vi "Test List Folder.vi"(8 "error in (no error)":errorcluster) -> (0 "error out":errorcluster, 3 "Pass?":bool)   [LabVIEW 2020]
uses:
  G-Unicode/Types/UTF-8 String/UTF-8 String.lvclass
  G-Unicode/Types/UTF-8 String/UTF-8 String.lvclass/UTF-8 String.ctl
  G-Unicode/Types/UTF-8 Path/UTF-8 Path.lvclass/UTF-8 Path.ctl
  a54f53b9-e182-45f2-9df3-3ad09404b159.vi
  2400d2f7-f357-4396-a7fa-e5c669c64687.vi
  2b28c85d-6eb6-42f1-9791-7ceb4d579ff7.vi
  8ef4e441-2967-427c-b2f5-611982e59b74.vi
  d10c2814-85e2-4189-8dec-6298f27de2e3.vi
  570365af-4a81-404b-8e59-15630106fe67.vi
  eeafece5-71ef-472f-ba41-926d6844275a.vi
  410ed48b-bd58-4d2b-973d-16e07af476d5.vi
  G-Unicode/Private/Conversion/Text as Encoded Path.vi
  G-Unicode/Private/Conversion/Polymorphic VIs/Text as Encoded Path (LabVIEW Path).vi
  G-Unicode/Types/UTF-8 Path/Write Encoded UTF-8 Path.vi
  G-Unicode/Private/Conversion/Path as Encoded Path.vi
  G-Unicode/Private/Conversion/Polymorphic VIs/Path as Encoded Path (LabVIEW Path).vi
  G-Unicode/Private/Conversion/Path as UTF-8 Path.vi
  G-Unicode/Private/Conversion/Polymorphic VIs/Path as UTF-8 Path (UTF-8 Path).vi
  2400d2f7-f357-4396-a7fa-e5c669c64687.vi/5269e09c-4216-478e-8686-9fb7d38e224a.vi
  2400d2f7-f357-4396-a7fa-e5c669c64687.vi/d1f4a45d-6f02-44dd-a40b-2b28d80e6519.vi
  G-Unicode/Private/Conversion/String as Encoded String.vi
  G-Unicode/Private/Conversion/Polymorphic VIs/String as Encoded String (UTF-8 String).vi
  G-Unicode/Private/Library/gu_list_folder.vi
  2400d2f7-f357-4396-a7fa-e5c669c64687.vi/8eb4f0ed-0012-4550-978e-be3f7301df70.vi
  2400d2f7-f357-4396-a7fa-e5c669c64687.vi/f7e6584c-01ed-423f-9bcd-660954191d0d.vi
  G-Unicode/Private/Conversion/Polymorphic VIs/Text as Encoded Path (UTF-8 String).vi
  G-Unicode/Private/Conversion/Polymorphic VIs/Path as Encoded Path (UTF-8 Path).vi
  8ef4e441-2967-427c-b2f5-611982e59b74.vi/5269e09c-4216-478e-8686-9fb7d38e224a.vi
  8ef4e441-2967-427c-b2f5-611982e59b74.vi/d1f4a45d-6f02-44dd-a40b-2b28d80e6519.vi
  8ef4e441-2967-427c-b2f5-611982e59b74.vi/8eb4f0ed-0012-4550-978e-be3f7301df70.vi
  8ef4e441-2967-427c-b2f5-611982e59b74.vi/f7e6584c-01ed-423f-9bcd-660954191d0d.vi
  570365af-4a81-404b-8e59-15630106fe67.vi/c24c063b-f849-48a1-b323-238a063d7118.vi
  570365af-4a81-404b-8e59-15630106fe67.vi/a2fd6c11-d594-45c9-8624-1f0a1df69df3.vi
  570365af-4a81-404b-8e59-15630106fe67.vi/1fd3173e-d32e-42cb-8f0d-819132eb8e27.vi
  570365af-4a81-404b-8e59-15630106fe67.vi/bb7c39fc-ad8e-447d-bc50-468674bfb562.vi
  G-Unicode/Private/Conversion/Polymorphic VIs/Path as UTF-8 Path (LabVIEW Path).vi
  eeafece5-71ef-472f-ba41-926d6844275a.vi/5269e09c-4216-478e-8686-9fb7d38e224a.vi
  eeafece5-71ef-472f-ba41-926d6844275a.vi/d1f4a45d-6f02-44dd-a40b-2b28d80e6519.vi
  eeafece5-71ef-472f-ba41-926d6844275a.vi/8eb4f0ed-0012-4550-978e-be3f7301df70.vi
  eeafece5-71ef-472f-ba41-926d6844275a.vi/f7e6584c-01ed-423f-9bcd-660954191d0d.vi
  G-Unicode/Private/Conversion/Polymorphic VIs/String as Encoded String (LabVIEW String).vi
  410ed48b-bd58-4d2b-973d-16e07af476d5.vi/5269e09c-4216-478e-8686-9fb7d38e224a.vi
  410ed48b-bd58-4d2b-973d-16e07af476d5.vi/d1f4a45d-6f02-44dd-a40b-2b28d80e6519.vi
  410ed48b-bd58-4d2b-973d-16e07af476d5.vi/8eb4f0ed-0012-4550-978e-be3f7301df70.vi
  410ed48b-bd58-4d2b-973d-16e07af476d5.vi/f7e6584c-01ed-423f-9bcd-660954191d0d.vi
  G-Unicode/Private/Conversion/Text to UTF-8.vi
  G-Unicode/Private/Conversion/Polymorphic VIs/Text to UTF-8 (LabVIEW Path).vi
  2400d2f7-f357-4396-a7fa-e5c669c64687.vi/5269e09c-4216-478e-8686-9fb7d38e224a.vi/c24c063b-f849-48a1-b323-238a063d7118.vi
  2400d2f7-f357-4396-a7fa-e5c669c64687.vi/5269e09c-4216-478e-8686-9fb7d38e224a.vi/a2fd6c11-d594-45c9-8624-1f0a1df69df3.vi
  2400d2f7-f357-4396-a7fa-e5c669c64687.vi/5269e09c-4216-478e-8686-9fb7d38e224a.vi/1fd3173e-d32e-42cb-8f0d-819132eb8e27.vi
  2400d2f7-f357-4396-a7fa-e5c669c64687.vi/5269e09c-4216-478e-8686-9fb7d38e224a.vi/bb7c39fc-ad8e-447d-bc50-468674bfb562.vi
  G-Unicode/Private/Conversion/Text as Encoded String.vi
  G-Unicode/Private/Conversion/Polymorphic VIs/Text as Encoded String (UTF-8 Path).vi
  2400d2f7-f357-4396-a7fa-e5c669c64687.vi/8eb4f0ed-0012-4550-978e-be3f7301df70.vi/3a31b270-3bb6-4c58-a256-c5fcc2c98f09.vi
  2400d2f7-f357-4396-a7fa-e5c669c64687.vi/8eb4f0ed-0012-4550-978e-be3f7301df70.vi/0ec5df2d-ef9b-4f84-a6a8-ffcedd45c4dc.vi
  G-Unicode/Private/Conversion/Text as String.vi
  G-Unicode/Private/Conversion/Polymorphic VIs/Text as String (UTF-8 Path).vi
  G-Unicode/Types/UTF-8 Path/Read Encoded UTF-8 Path.vi
  8ef4e441-2967-427c-b2f5-611982e59b74.vi/5269e09c-4216-478e-8686-9fb7d38e224a.vi/c24c063b-f849-48a1-b323-238a063d7118.vi
  8ef4e441-2967-427c-b2f5-611982e59b74.vi/5269e09c-4216-478e-8686-9fb7d38e224a.vi/a2fd6c11-d594-45c9-8624-1f0a1df69df3.vi
  8ef4e441-2967-427c-b2f5-611982e59b74.vi/5269e09c-4216-478e-8686-9fb7d38e224a.vi/1fd3173e-d32e-42cb-8f0d-819132eb8e27.vi
  8ef4e441-2967-427c-b2f5-611982e59b74.vi/5269e09c-4216-478e-8686-9fb7d38e224a.vi/bb7c39fc-ad8e-447d-bc50-468674bfb562.vi
  8ef4e441-2967-427c-b2f5-611982e59b74.vi/8eb4f0ed-0012-4550-978e-be3f7301df70.vi/3a31b270-3bb6-4c58-a256-c5fcc2c98f09.vi
  8ef4e441-2967-427c-b2f5-611982e59b74.vi/8eb4f0ed-0012-4550-978e-be3f7301df70.vi/0ec5df2d-ef9b-4f84-a6a8-ffcedd45c4dc.vi
  G-Unicode/Private/Library/gu_string_subset.vi
  G-Unicode/Private/Library/gu_to_lower_case.vi
  G-Unicode/Private/Library/gu_search_split_string.vi
  G-Unicode/Types/UTF-8 Path/New UTF-8 Path.vi
  eeafece5-71ef-472f-ba41-926d6844275a.vi/5269e09c-4216-478e-8686-9fb7d38e224a.vi/c24c063b-f849-48a1-b323-238a063d7118.vi
  eeafece5-71ef-472f-ba41-926d6844275a.vi/5269e09c-4216-478e-8686-9fb7d38e224a.vi/a2fd6c11-d594-45c9-8624-1f0a1df69df3.vi
  eeafece5-71ef-472f-ba41-926d6844275a.vi/5269e09c-4216-478e-8686-9fb7d38e224a.vi/1fd3173e-d32e-42cb-8f0d-819132eb8e27.vi
  eeafece5-71ef-472f-ba41-926d6844275a.vi/5269e09c-4216-478e-8686-9fb7d38e224a.vi/bb7c39fc-ad8e-447d-bc50-468674bfb562.vi
  eeafece5-71ef-472f-ba41-926d6844275a.vi/8eb4f0ed-0012-4550-978e-be3f7301df70.vi/3a31b270-3bb6-4c58-a256-c5fcc2c98f09.vi
  eeafece5-71ef-472f-ba41-926d6844275a.vi/8eb4f0ed-0012-4550-978e-be3f7301df70.vi/0ec5df2d-ef9b-4f84-a6a8-ffcedd45c4dc.vi
  G-Unicode/Private/Conversion/Polymorphic VIs/Text to UTF-8 (LabVIEW String).vi
  410ed48b-bd58-4d2b-973d-16e07af476d5.vi/5269e09c-4216-478e-8686-9fb7d38e224a.vi/c24c063b-f849-48a1-b323-238a063d7118.vi
  410ed48b-bd58-4d2b-973d-16e07af476d5.vi/5269e09c-4216-478e-8686-9fb7d38e224a.vi/a2fd6c11-d594-45c9-8624-1f0a1df69df3.vi
  410ed48b-bd58-4d2b-973d-16e07af476d5.vi/5269e09c-4216-478e-8686-9fb7d38e224a.vi/1fd3173e-d32e-42cb-8f0d-819132eb8e27.vi
  410ed48b-bd58-4d2b-973d-16e07af476d5.vi/5269e09c-4216-478e-8686-9fb7d38e224a.vi/bb7c39fc-ad8e-447d-bc50-468674bfb562.vi
  410ed48b-bd58-4d2b-973d-16e07af476d5.vi/8eb4f0ed-0012-4550-978e-be3f7301df70.vi/3a31b270-3bb6-4c58-a256-c5fcc2c98f09.vi
  410ed48b-bd58-4d2b-973d-16e07af476d5.vi/8eb4f0ed-0012-4550-978e-be3f7301df70.vi/0ec5df2d-ef9b-4f84-a6a8-ffcedd45c4dc.vi
  G-Unicode/Private/Conversion/Polymorphic VIs/Text as Encoded String (UTF-8 String).vi
  G-Unicode/Private/Conversion/Polymorphic VIs/Text as Encoded String (LabVIEW String).vi
  G-Unicode/Private/Memory/Copy String.vi
  G-Unicode/Private/Memory/Copy String.vi/4d47babd-4a2d-4eb7-b91b-7e707d692665.vi
  G-Unicode/Private/Library/gu_free.vi
  G-Unicode/Unicode/Detect String Encoding.vi
  G-Unicode/Private/Conversion/Encoded UTF-16LE String to Encoded UTF-8 String.vi
  G-Unicode/Private/Memory/Copy String Array.vi
  G-Unicode/File IO/Path to Short Name.vi
  G-Unicode/Types/UTF-8 Path/UTF-8 Path.lvclass
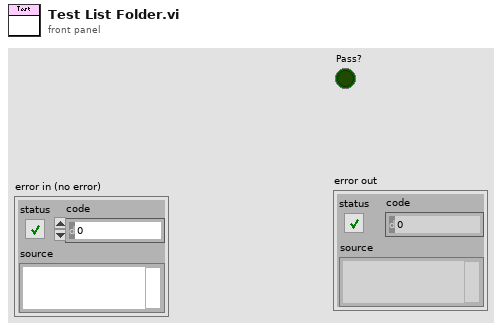
[diagram p1: front panel]
types:
  T1 = typedef "G-Unicode.lvlib/Encoded UTF-8 String.ctl" = string
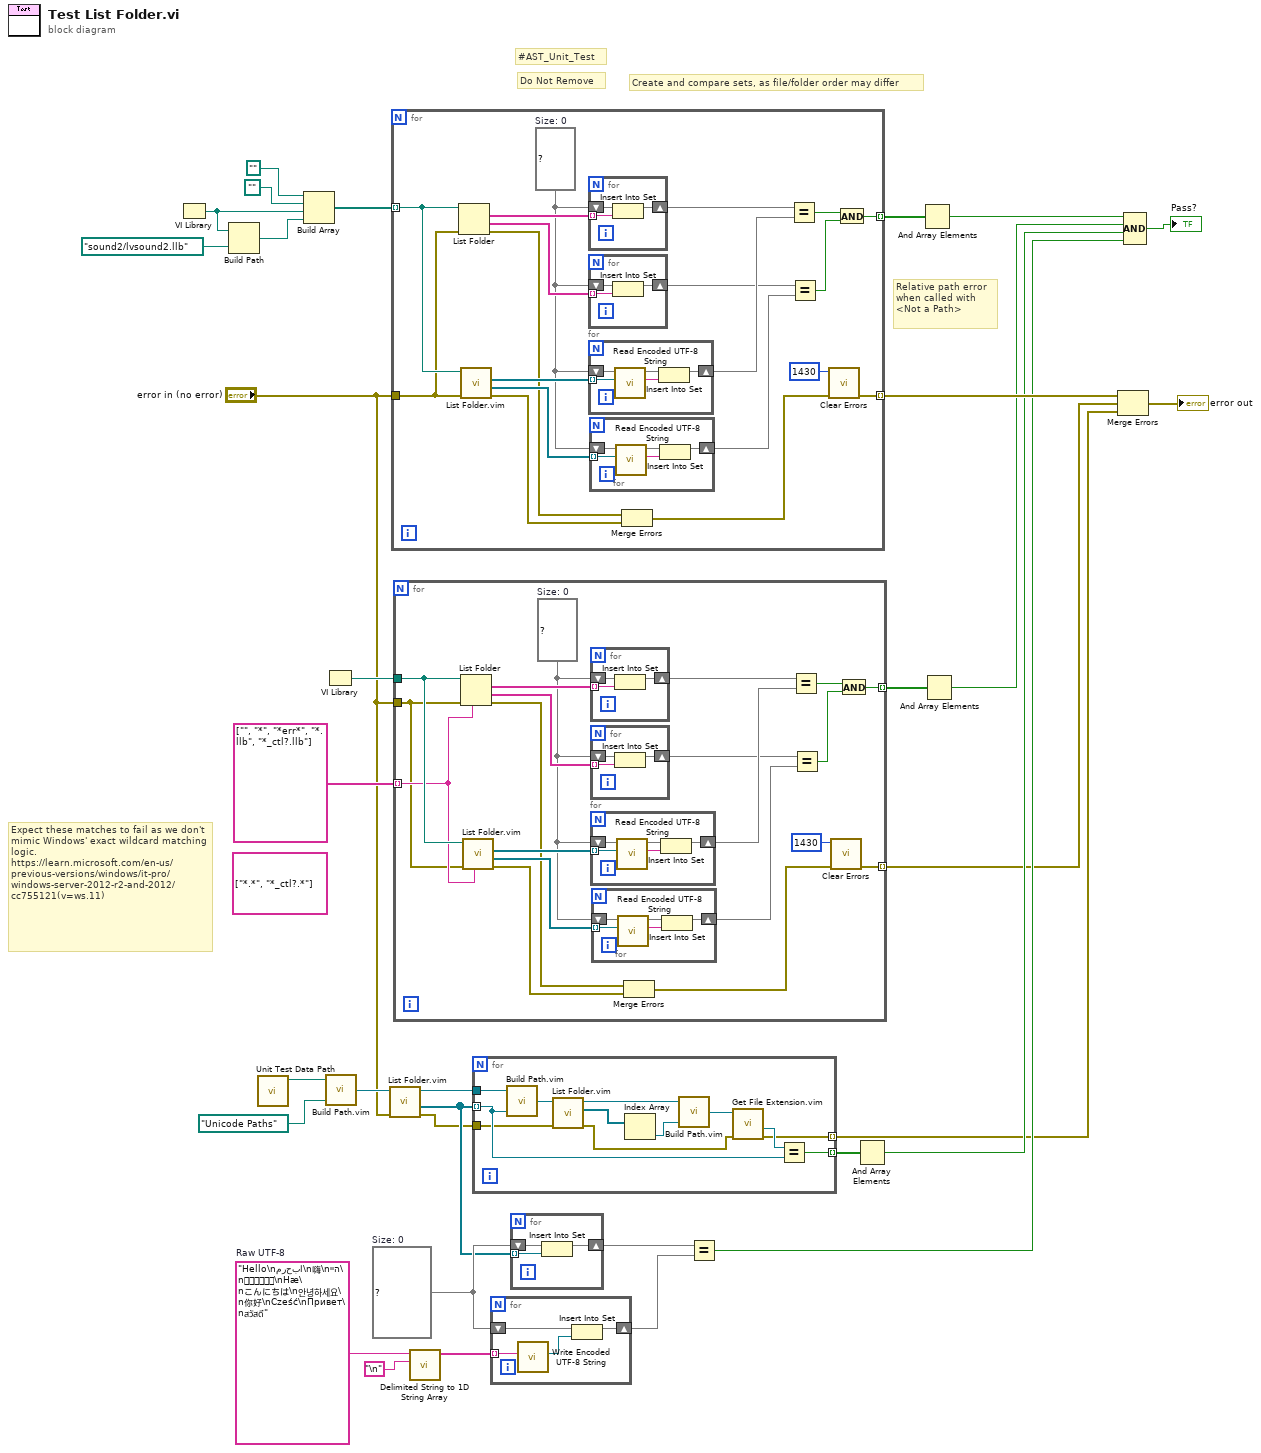
[diagram p0: block diagram]
diagram:
  (unwired) string[] ["*.*", "*_ctl?.*"]
  w23 = set{refnum<class "UTF-8 String.lvclass">} {}  # Size: 0
  w25 = "Hello\nمرحبا\n嗨\nהיי\nनमस्ते\nHæ\nこんにちは\n안녕하세요\n你好\nCześć\nПривет\nสวัสดี"  # Raw UTF-8
  # "Expect these matches to fail as we don't mimic Windows' exact wildcard matching logic.\nhttps://learn.microsoft.com/en-us/previous-versions/windows/it-pro/windows-server-2012-r2-and-2012/cc755121(v=ws.11)"
  # "Create and compare sets, as file/folder order may differ"
  # "Relative path error when called with <Not a Path>"
  # "Do Not Remove"
  # "#AST_Unit_Test"
  n1 = VI Library() -> (path=w9:path)
  n2 = Build Path(base path=w9, name or relative path=path "sound2/lvsound2.llb") -> (appended path=w10:path)
  n3 = call "Unit Test Data Path.vi"() -> ("Test Data Path"=w18:path)  [unwired: 11 in]
  n4 = Build Array(path "", path "", w9, w10) -> (w31:path[])
  n5 = VI Library() -> (path=w7:path)
  n6 = call "Build Path.vim"("Base Path"=w18, "Name or Relative Path"=path "Unicode Paths") -> ("Appended Path"=w17:refnum<class "UTF-8 Path.lvclass">)  [unwired: 6 in, 1 out]
  n7 = call "List Folder.vim"("error in"="error in (no error)", "Path"=w17) -> ("error out"=w2:errorcluster, "Folder Names"=w15:refnum<class "UTF-8 String.lvclass">[], "Path Out"=w14:refnum<class "UTF-8 Path.lvclass">)  [unwired: 6 in, 1 out]
  n8 = for {
    tunnel: w31 -> [w52] mode=indexing
    tunnel: [w39] -> w33 mode=indexing
    tunnel: "error in (no error)" -> [w49]
    tunnel: [w35] -> w32 mode=indexing
    w46 = set{string} {}  # Size: 0
    n9 = List Folder(path=w52, error in=w49) -> (filenames=w51:string[], folder names=w50:string[], error out=w38:errorcluster)  [unwired: 2 in, 1 out]
    n10 = call "List Folder.vim"("error in"=w49, "Path"=w52) -> ("error out"=w37:errorcluster, "Folder Names"=w47:refnum<class "UTF-8 String.lvclass">[], "Filenames"=w48:refnum<class "UTF-8 String.lvclass">[])  [unwired: 6 in, 1 out]
    n11 = for {
      tunnel: w51 -> [w66] mode=indexing
      shift-right: [w64] -> w45
      shift-left: w46 -> [w65]
      n12 = Insert Into Set(10:w66, 11:w65) -> (3:w64:set{string})  [unwired: 1 out]
    }
    n13 = for {
      tunnel: w50 -> [w63] mode=indexing
      shift-right: [w61] -> w43
      shift-left: w46 -> [w62]
      n14 = Insert Into Set(10:w63, 11:w62) -> (3:w61:set{string})  [unwired: 1 out]
    }
    n15 = for {
      tunnel: w48 -> [w58] mode=indexing
      shift-right: [w59] -> w44
      shift-left: w46 -> [w60]
      n16 = call "Read Encoded UTF-8 String.vi"("UTF-8 String"=w58) -> ("Encoded UTF-8 String"=w57:T1)  [unwired: 10 in]
      n17 = Insert Into Set(10:w57, 11:w60) -> (3:w59:set{string})  [unwired: 1 out]
    }
    n18 = for {
      tunnel: w47 -> [w54] mode=indexing
      shift-right: [w55] -> w42
      shift-left: w46 -> [w56]
      n19 = call "Read Encoded UTF-8 String.vi"("UTF-8 String"=w54) -> ("Encoded UTF-8 String"=w53:T1)  [unwired: 10 in]
      n20 = Insert Into Set(10:w53, 11:w56) -> (3:w55:set{string})  [unwired: 1 out]
    }
    n21 = Merge Errors(w38, w37) -> (w36:errorcluster)
    n22 = Equal?(x=w45, y=w44) -> (x = y?=w41:bool)
    n23 = Equal?(x=w43, y=w42) -> (x = y?=w40:bool)
    n24 = call <vilib>:"Clear Errors.vi"("error in (no error)"=w36, "specific error code to clear (0: all)"=1430) -> ("error out"=w35:errorcluster)  [unwired: 4 in, 1 out]
    n25 = And(x=w41, y=w40) -> (x .and. y?=w39:bool)
  }
  n26 = for {
    tunnel: w7 -> [w86]
    tunnel: [w74] -> w8 mode=indexing
    tunnel: [w70] -> w4 mode=indexing
    tunnel: string[] ["", "*", "*err*", "*.llb", "*_ctl?.llb"] -> [w68] mode=indexing
    tunnel: "error in (no error)" -> [w67]
    w81 = set{string} {}  # Size: 0
    n27 = List Folder(path=w86, pattern=w68, error in=w67) -> (filenames=w85:string[], folder names=w84:string[], error out=w73:errorcluster)  [unwired: 1 in, 1 out]
    n28 = call "List Folder.vim"("Pattern"=w68, "error in"=w67, "Path"=w86) -> ("error out"=w72:errorcluster, "Folder Names"=w82:refnum<class "UTF-8 String.lvclass">[], "Filenames"=w83:refnum<class "UTF-8 String.lvclass">[])  [unwired: 5 in, 1 out]
    n29 = for {
      tunnel: w85 -> [w100] mode=indexing
      shift-right: [w98] -> w80
      shift-left: w81 -> [w99]
      n30 = Insert Into Set(10:w100, 11:w99) -> (3:w98:set{string})  [unwired: 1 out]
    }
    n31 = for {
      tunnel: w84 -> [w97] mode=indexing
      shift-right: [w95] -> w78
      shift-left: w81 -> [w96]
      n32 = Insert Into Set(10:w97, 11:w96) -> (3:w95:set{string})  [unwired: 1 out]
    }
    n33 = for {
      tunnel: w83 -> [w92] mode=indexing
      shift-right: [w93] -> w79
      shift-left: w81 -> [w94]
      n34 = call "Read Encoded UTF-8 String.vi"("UTF-8 String"=w92) -> ("Encoded UTF-8 String"=w91:T1)  [unwired: 10 in]
      n35 = Insert Into Set(10:w91, 11:w94) -> (3:w93:set{string})  [unwired: 1 out]
    }
    n36 = for {
      tunnel: w82 -> [w88] mode=indexing
      shift-right: [w89] -> w77
      shift-left: w81 -> [w90]
      n37 = call "Read Encoded UTF-8 String.vi"("UTF-8 String"=w88) -> ("Encoded UTF-8 String"=w87:T1)  [unwired: 10 in]
      n38 = Insert Into Set(10:w87, 11:w90) -> (3:w89:set{string})  [unwired: 1 out]
    }
    n39 = Merge Errors(w73, w72) -> (w71:errorcluster)
    n40 = Equal?(x=w80, y=w79) -> (x = y?=w76:bool)
    n41 = Equal?(x=w78, y=w77) -> (x = y?=w75:bool)
    n42 = call <vilib>:"Clear Errors.vi"("error in (no error)"=w71, "specific error code to clear (0: all)"=1430) -> ("error out"=w70:errorcluster)  [unwired: 4 in, 1 out]
    n43 = And(x=w76, y=w75) -> (x .and. y?=w74:bool)
  }
  n44 = call <vilib>:"Delimited String to 1D String Array.vi"("delimiter"="\n", "delimited string"=w25) -> ("string array"=w24:string[])  [unwired: 9 in]
  n45 = for {
    tunnel: w15 -> [w105] mode=indexing
    tunnel: w14 -> [w112]
    tunnel: [w104] -> w13 mode=indexing
    tunnel: w2 -> [w103]
    tunnel: [w101] -> w3 mode=indexing
    n46 = call "Build Path.vim"("Base Path"=w112, "Name or Relative Path"=w105) -> ("Appended Path"=w111:refnum<class "UTF-8 Path.lvclass">)  [unwired: 6 in, 1 out]
    n47 = call "List Folder.vim"("error in"=w103, "Path"=w111) -> ("error out"=w102:errorcluster, "Filenames"=w110:refnum<class "UTF-8 String.lvclass">[], "Path Out"=w109:refnum<class "UTF-8 Path.lvclass">)  [unwired: 6 in, 1 out]
    n48 = Index Array(array=w110) -> (element=w108:refnum<class "UTF-8 String.lvclass">)  [unwired: 1 in]
    n49 = call "Build Path.vim"("Base Path"=w109, "Name or Relative Path"=w108) -> ("Appended Path"=w107:refnum<class "UTF-8 Path.lvclass">)  [unwired: 6 in, 1 out]
    n50 = call "Get File Extension.vim"("error in (no error)"=w102, "file"=w107) -> ("error out"=w101:errorcluster, "filename without extension"=w106:refnum<class "UTF-8 String.lvclass">)  [unwired: 5 in, 3 out]
    n51 = Equal?(x=w106, y=w105) -> (x = y?=w104:bool)
  }
  n52 = for {
    tunnel: w24 -> [w114] mode=indexing
    shift-right: [w115] -> w21
    shift-left: w23 -> [w116]
    n53 = call "Write Encoded UTF-8 String.vi"("Encoded UTF-8 String"=w114) -> ("UTF-8 String"=w113:refnum<class "UTF-8 String.lvclass">)  [unwired: 10 in]
    n54 = Insert Into Set(10:w113, 11:w116) -> (3:w115:set{refnum<class "UTF-8 String.lvclass">})  [unwired: 1 out]
  }
  n55 = for {
    tunnel: w15 -> [w117] mode=indexing
    shift-right: [w118] -> w22
    shift-left: w23 -> [w119]
    n56 = Insert Into Set(10:w117, 11:w119) -> (3:w118:set{refnum<class "UTF-8 String.lvclass">})  [unwired: 1 out]
  }
  n57 = Equal?(x=w22, y=w21) -> (x = y?=w12:bool)
  n58 = And Array Elements(Boolean array=w13) -> (logical AND=w11:bool)
  n59 = And Array Elements(Boolean array=w33) -> (logical AND=w20:bool)
  n60 = And Array Elements(Boolean array=w8) -> (logical AND=w5:bool)
  n61 = Merge Errors(w32, w4, w3) -> (→"error out":errorcluster)
  n62 = Compound Arithmetic op=AND(w20, w5, w11, w12) -> (→"Pass?":bool)
